vi "Eurotherm - Generate Checksum.vi"(0 "String":string) -> (4 "Checksum Character":string, 8 "Checksum Number":u8)   [LabVIEW 2011]
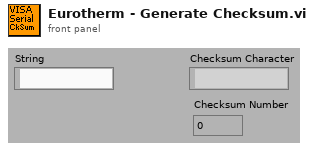
[diagram p1: front panel]
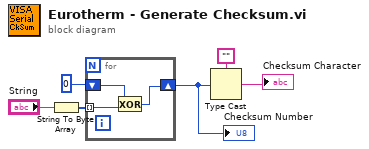
[diagram p0: block diagram]
diagram:
  n1 = String To Byte Array(string="String") -> (unsigned byte array=w5:u8[])
  n2 = for {
    shift-right: [w8] -> w1
    shift-left: u8 0 -> [w9]
    tunnel: w5 -> [w7] mode=indexing
    n3 = Exclusive Or(1:w7, 2:w9) -> (0:w8:u8)
  }
  "Checksum Number" <- w1
  n4 = Type Cast(type="", x=w1) -> (*(type *) &x=→"Checksum Character":string)
